vi "Main VI.vi"() -> ()   [LabVIEW 2011]
doc: "Use this template to build a producer/consumer design pattern with events to produce queue items. Use this design pattern instead of the User Interface Event Handler pattern for user interfaces when you want to execute code asynchronously in response to an event without slowing the user interface responsiveness."
uses:
  Event FGV Actions.ctl
panel:
  out "Timer Before Dynamic User Event":u8(slide)=4 scale=0.0..10.0
  out "Data Received":string
  in  "Any string to pass dynamically":string="Dynamic User Event"
  in  "Enqueue Element":bool
  in  "stop":bool
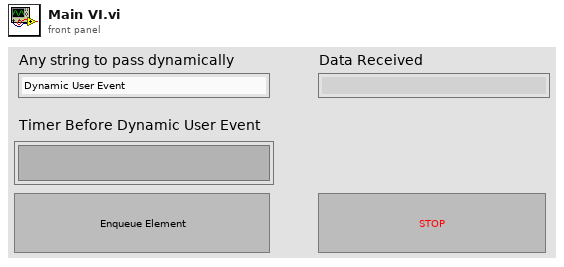
[diagram p1: front panel]
types:
  T1 = typedef "Event FGV Actions.ctl" = enum16{"Register Event", "Fire Event"}
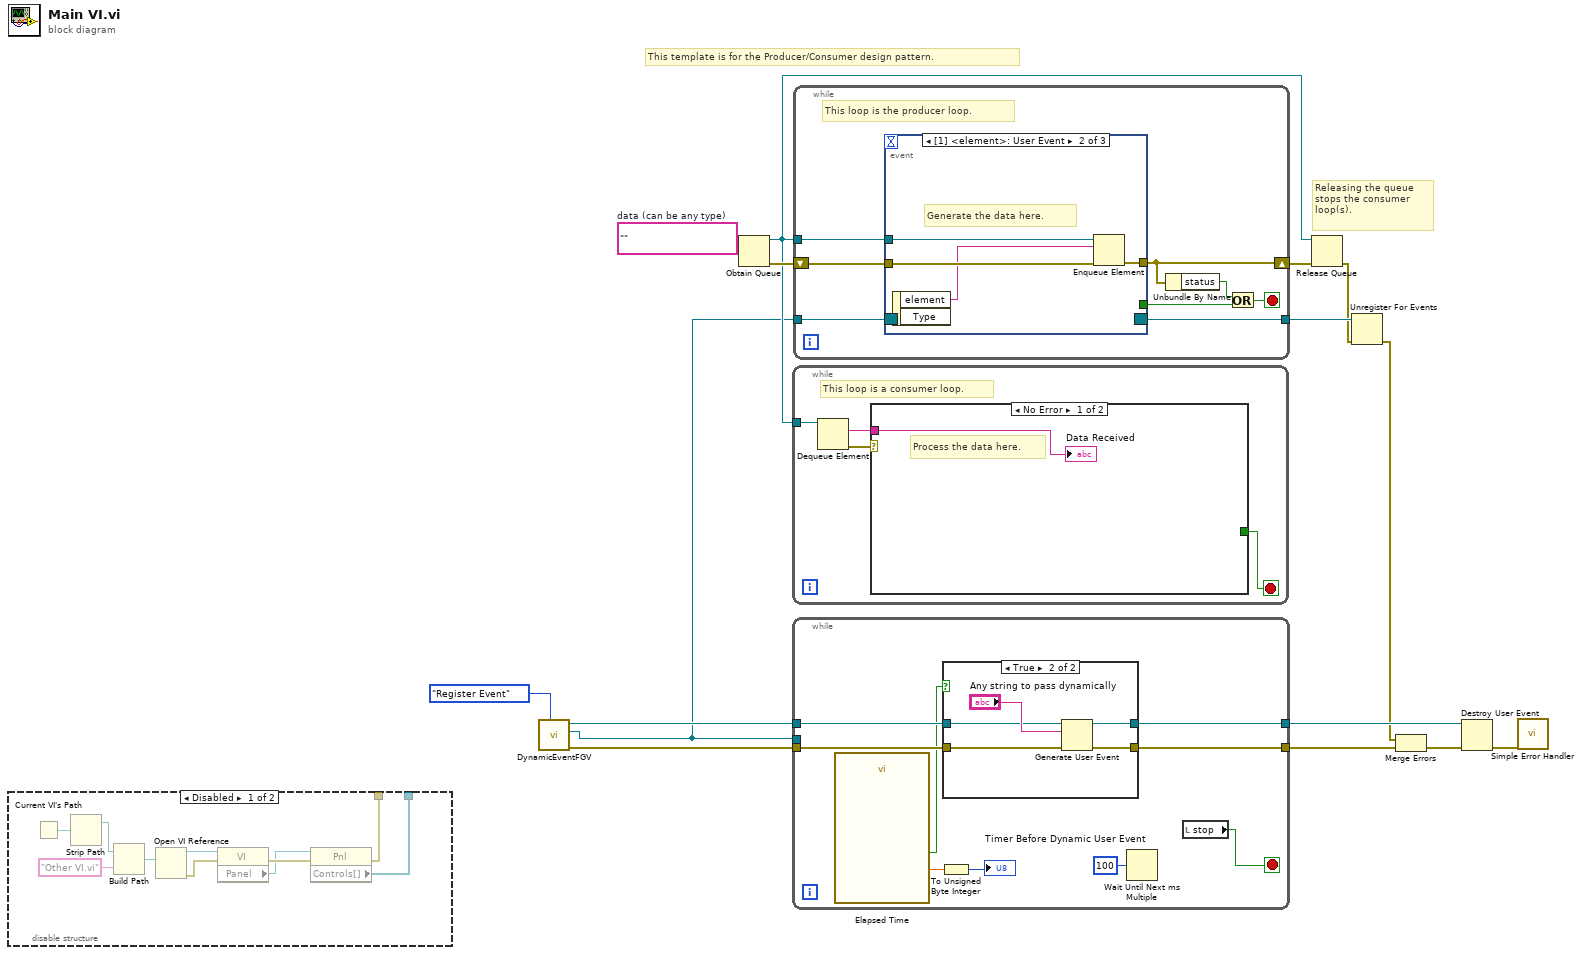
[diagram p0: block diagram]
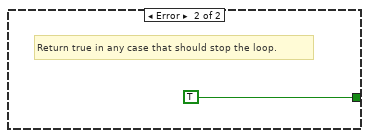
[diagram p4: hidden frame]
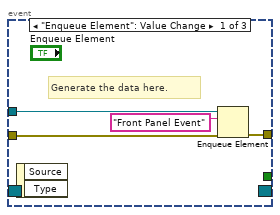
[diagram p5: hidden frame]
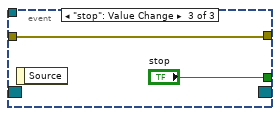
[diagram p6: hidden frame]
diagram:
  w13 = ""  # data (can be any type)
  # "Releasing the queue stops the consumer loop(s)."
  # "This template is for the Producer/Consumer design pattern."
  n1 = disable-structure shown="Disabled" {
    disable-tunnel: [w23 _] -> _
    disable-tunnel: [w20 _] -> _
    frame Disabled {
      n2 = Current VI's Path() -> (path=w17:path)
      n3 = Strip Path(path=w17) -> (stripped path=w16:path)  [unwired: 1 out]
      n4 = Build Path(base path=w16, name or relative path="Other VI.vi") -> (appended path=w19:path)
      n5 = Open VI Reference(vi path=w19) -> (vi reference=w22:refnum<vi>, error out=w25:errorcluster)  [unwired: 5 in]
      n6 = property class="VI"(reference=w22, error in=w25) -> (error out=w24:errorcluster, "Panel"=w21:refnum<vi>)  [unwired: 1 out]
      n7 = property class="Pnl"(reference=w21, error in=w24) -> (error out=w20:errorcluster, "Controls[]"=w23:refnum<vi>[])  [unwired: 1 out]
    }
    frame Enabled {
    }
  }
  n8 = call "DynamicEventFGV.vi"("Event FGV Actions"=Event_FGV_Actions."Register Event") -> ("error out"=w4:errorcluster, "Event Registration Refnum"=w2:refnum<event-registration>, "element"=w3:refnum<user-event>)  [unwired: 8 in]
  n9 = Obtain Queue(element data type=w13) -> (queue out=w12:refnum<queue>, error out=w15:errorcluster)  [unwired: 4 in, 1 out]
  n10 = while {
    tunnel: w12 -> [w29]
    stop <- w26 stop-if-true
    # "This loop is a consumer loop."
    n11 = Dequeue Element(queue=w29) -> (element=w27:string, error out=w28:errorcluster)  [unwired: 2 in, 2 out]
    n12 = case shown="No Error" w28 {
      tunnel: w27 -> [w30 _]
      tunnel: [_ TRUE] -> w26
      frame No Error {
        # "Process the data here."
        "Data Received" <- w30
      }
      frame Error {
        # "Return true in any case that should stop the loop."
      }
    }
  }
  n13 = while {
    tunnel: w2 -> [_]
    tunnel: w4 -> [w40]
    tunnel: [w39] -> w8
    tunnel: w3 -> [w38]
    tunnel: [w37] -> w9
    stop <- w32 stop-if-true
    n14 = call "Elapsed Time"() -> ("Elapsed Time (s)"=w34:dbl, "Time has Elapsed"=w36:bool)  [unwired: 12 in, 6 out]
    n15 = To Unsigned Byte Integer(number=w34) -> (unsigned 8bit integer=→"Timer Before Dynamic User Event":u8)
    n16 = case shown="True" w36 {
      tunnel: w40 -> [w41 w47]
      tunnel: [w41 w45] -> w39
      tunnel: w38 -> [w42 w44]
      tunnel: [w42 w43] -> w37
      frame False {
      }
      frame True {
        n17 = Generate User Event(user event=w44, event data cluster="Any string to pass dynamically", error in=w47) -> (user event out=w43:refnum<user-event>, error out=w45:errorcluster)
      }
    }
    n18 = Wait Until Next ms Multiple(millisecond multiple=u32 100) -> ()  [unwired: 1 out]
    n19 = local read "stop"() -> (w32:bool)
  }
  n20 = while {
    shift-right: [w51] -> w14
    shift-left: w15 -> [w54]
    tunnel: w12 -> [w55]
    tunnel: w2 -> [w49]
    tunnel: [w48] -> w11
    stop <- w52 stop-if-true
    # "This loop is the producer loop."
    n21 = event shown="[1] <element>: User Event" {
      selector: w49 -> [_ _ _]
      dyn-events: [_ _ _] -> w48
      timeout: _ -> [_ _ _]
      tunnel: w55 -> [w59 w63 _]
      tunnel: w54 -> [w58 w62 w64]
      tunnel: [w57 w61 w64] -> w51
      tunnel: [_ _ "stop"] -> w53
      event "Enqueue Element": Value Change {
        # "Generate the data here."
        n22 = event-data() -> ()  [unwired: 1 in, 2 out]
        n23 = Enqueue Element(queue=w59, element="Front Panel Event", error in (no error)=w58) -> (error out=w57:errorcluster)  [unwired: 1 in, 2 out]
      }
      event User Event {
        # "Generate the data here."
        n24 = event-data() -> ("element"=w60:string)  [unwired: 1 in, 1 out]
        n25 = Enqueue Element(queue=w63, element=w60, error in (no error)=w62) -> (error out=w61:errorcluster)  [unwired: 1 in, 2 out]
      }
      event "stop": Value Change {
        n26 = event-data() -> ()  [unwired: 1 in, 1 out]
      }
    }
    n27 = Unbundle By Name(w51) -> ("status"=w50:bool)
    n28 = Or(x=w50, y=w53) -> (x .or. y?=w52:bool)
  }
  n29 = Release Queue(queue=w12, error in (no error)=w14) -> (error out=w10:errorcluster)  [unwired: 1 in, 2 out]
  n30 = Unregister For Events(event registration refnum=w11, error in=w10) -> (error out=w7:errorcluster)
  n31 = Merge Errors(w7, w8) -> (w6:errorcluster)
  n32 = Destroy User Event(user event=w9, error in=w6) -> (error out=w5:errorcluster)
  n33 = call <vilib>:"Simple Error Handler.vi"("error in (no error)"=w5) -> ()  [unwired: 4 in, 5 out]
